vi "Write Run Url File.vi"(8 "Sift Client in":refnum<class "Sift Client.lvclass">, 9 "error in (no error)":errorcluster, 10 "TDMS Filepath":path, 11 "Run URL":string) -> ()   [LabVIEW 2024, in "Sift TDMS Uploader.lvlib" / "Sift TDMS Uploader.lvclass"]
uses:
  Sift TDMS Uploader.lvclass
  <vilib>/Sift/Sift/Sift API/Sift Client.lvclass
  <vilib>/Utility/config.llb/Write Key (String).vi
  Sift TDMS Uploader.lvclass/Sift TDMS Uploader.ctl
  <vilib>/Utility/config.llb/NI_LVConfig.lvlib
panel:
  out "error out":errorcluster
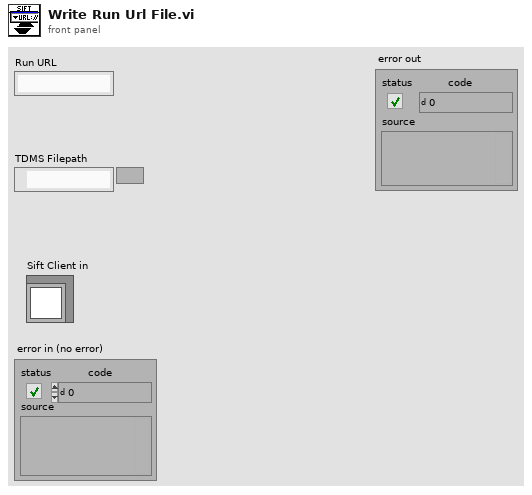
[diagram p1: front panel]
types:
  T1 = enum16{"open", "replace", "create", "open or create", "replace or create", "replace or create with confirmation"}
  T2 = typedef "NI_LVConfig.lvlib/Config Data RefNum.ctl" = refnum<k1>
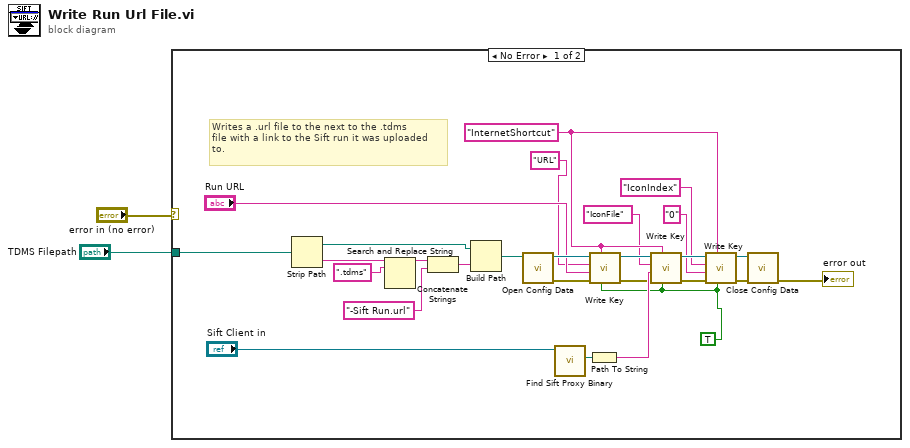
[diagram p0: block diagram]
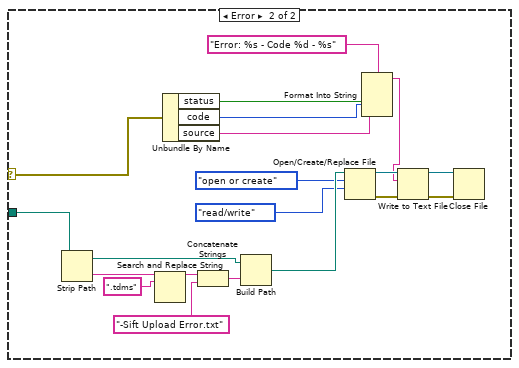
[diagram p2: hidden frame]
diagram:
  n1 = case shown="No Error" "error in (no error)" {
    selector: "error in (no error)" -> [_ w49]
    tunnel: "TDMS Filepath" -> [w3 w42]
    frame No Error {
      w11 = TRUE
      w10 = "InternetShortcut"
      # "Writes a .url file to the next to the .tdms\nfile with a link to the Sift run it was uploaded\nto."
      n2 = Strip Path(path=w3) -> (stripped path=w25:path, name=w24:string)
      n3 = Search and Replace String(input string=w24, search string=".tdms") -> (result string=w23:string)  [unwired: 6 in, 3 out]
      n4 = Concatenate Strings(w23, "-Sift Run.url") -> (w22:string)
      n5 = Build Path(base path=w25, name or relative path=w22) -> (appended path=w21:path)
      n6 = call <vilib>:"Open Config Data.vi"("configuration file path"=w21) -> ("error out"=w17:errorcluster, "refnum"=w20:T2)  [unwired: 8 in, 1 out]
      n7 = call-dynamic "Find Sift Proxy Binary.vi"("Sift Client in"="Sift Client in") -> ("Path"=w29:path)  [unwired: 7 in, 3 out]
      n8 = Path To String(path=w29) -> (string=w28:string)
      n9 = call-poly <vilib>:"Write Key.vi"("write raw string? (F)"=w11, "section"=w10, "error in (no error)"=w17, "value"="Run URL", "key"="URL", "refnum"=w20) -> ("error out"=w16:errorcluster, "refnum out"=w18:T2)  [unwired: 3 in, 1 out]
      n10 = call-poly <vilib>:"Write Key.vi"("write raw string? (F)"=w11, "section"=w10, "error in (no error)"=w16, "value"=w28, "key"="IconFile", "refnum"=w18) -> ("error out"=w15:errorcluster, "refnum out"=w14:T2)  [unwired: 3 in, 1 out]
      n11 = call-poly <vilib>:"Write Key.vi"("write raw string? (F)"=w11, "section"=w10, "error in (no error)"=w15, "value"="0", "key"="IconIndex", "refnum"=w14) -> ("error out"=w12:errorcluster, "refnum out"=w13:T2)  [unwired: 3 in, 1 out]
      n12 = call <vilib>:"Close Config Data.vi"("error in (no error)"=w12, "refnum"=w13) -> ("error out"=→"error out":errorcluster)  [unwired: 8 in, 1 out]
    }
    frame Error {
      n13 = Strip Path(path=w42) -> (stripped path=w48:path, name=w47:string)
      n14 = Search and Replace String(input string=w47, search string=".tdms") -> (result string=w46:string)  [unwired: 6 in, 3 out]
      n15 = Unbundle By Name(w49) -> ("status"=w32:bool, "code"=w30:i32, "source"=w31:string)
      n16 = Concatenate Strings(w46, "-Sift Upload Error.txt") -> (w45:string)
      n17 = Build Path(base path=w48, name or relative path=w45) -> (appended path=w41:path)
      n18 = Open/Create/Replace File(file path (use dialog)=w41, operation (0:open)=T1."open or create", access (0:read/write)=enum16{"read/write", "read-only", "write-only"}."read/write") -> (refnum out=w38:refnum<file>, error out=w36:errorcluster)  [unwired: 3 in, 1 out]
      n19 = Format Into String(format string="Error: %s - Code %d - %s", w32, w30, w31) -> (resulting string=w34:string)  [unwired: 2 in, 1 out]
      n20 = Write to Text File(file (use dialog)=w38, text=w34, error in=w36) -> (refnum out=w37:refnum<file>, error out=w35:errorcluster)  [unwired: 1 in, 1 out]
      n21 = Close File(refnum=w37, error in=w35) -> ()  [unwired: 2 out]
    }
  }
